vi "DriveStateController2.vi"(1 "Selected State (In)":string) -> (0 "Selected State (Out)":string)   [LabVIEW 2019]
doc: "This VI performs all of the calculations and decisions related to the swerve drive."
uses:
  dsinstructions.vi
  outputs.vi
  sensors.vi
  dsdata.vi
  constants.vi
panel:
  out "Heading Control":bool
  in  "Heading Lock Strafe Deadband (ft/s)":dbl=2.0
  in  "PID Tuning Heading Lock":T1={"Kp"=0.007, "Ki"=0.03, "Kd"=0.0015, "N-Diff"=5, "N-Int"=10, "Int Error Window"=30.0, "Max Ouput"=1.0, "Min Output"=-1.0} {"Int Error Window" min=0.0; "N-Int" min=2; "N-Diff" min=2; "Kd" min=0.0; "Ki" min=0.0; "Kp" min=0.0}
  in  "Manually Disable Heading Lock":bool
  in  "PID Tuning Feeder Station":T1={"Kp"=0.01, "Ki"=0.01, "Kd"=9e-05, "N-Diff"=10, "N-Int"=10, "Int Error Window"=30.0, "Max Ouput"=1.0, "Min Output"=-1.0} {"Int Error Window" min=0.0; "N-Int" min=2; "N-Diff" min=2; "Kd" min=0.0; "Ki" min=0.0; "Kp" min=0.0}
  out "Heading Controller Summary":T2(graph)
  in  "PID Tuning Auto Targeting":T1={"Kp"=0.01, "Ki"=0.01, "Kd"=9e-05, "N-Diff"=10, "N-Int"=10, "Int Error Window"=30.0, "Max Ouput"=1.0, "Min Output"=-1.0} {"Int Error Window" min=0.0; "N-Int" min=2; "N-Diff" min=2; "Kd" min=0.0; "Ki" min=0.0; "Kp" min=0.0}
  in  "Manual Fudge Factor (deg)":dbl=5.0
  in  "Plot Heading PID":bool
  in  "Rotation Scaling":dbl[](array[slide])=[2.5, 2.5, 2.5, 2.5] min=1.0 max=4.0 scale=1.0..4.0
  in  "Strafe Scaling":dbl[](array[slide])=[3.0, 2.0, 2.0, 2.0] min=1.0 max=4.0 scale=1.0..4.0
  in  "Rotation Deadband":dbl[](array[slide])=[0.15, 0.15, 0.15, 0.15] min=0.0 max=0.4 scale=0.0..0.4
  in  "Strafe Deadband":dbl[](array[slide])=[0.08, 0.08, 0.08, 0.08] min=0.0 max=0.4 scale=0.0..0.4
  in  "Sync Driver Profile":bool
  out "Current_Driver":string
  in  "Zero Wheels":bool
  in  "Best Angle Hysteresis (deg)":dbl=20.0 format="%#_13g"
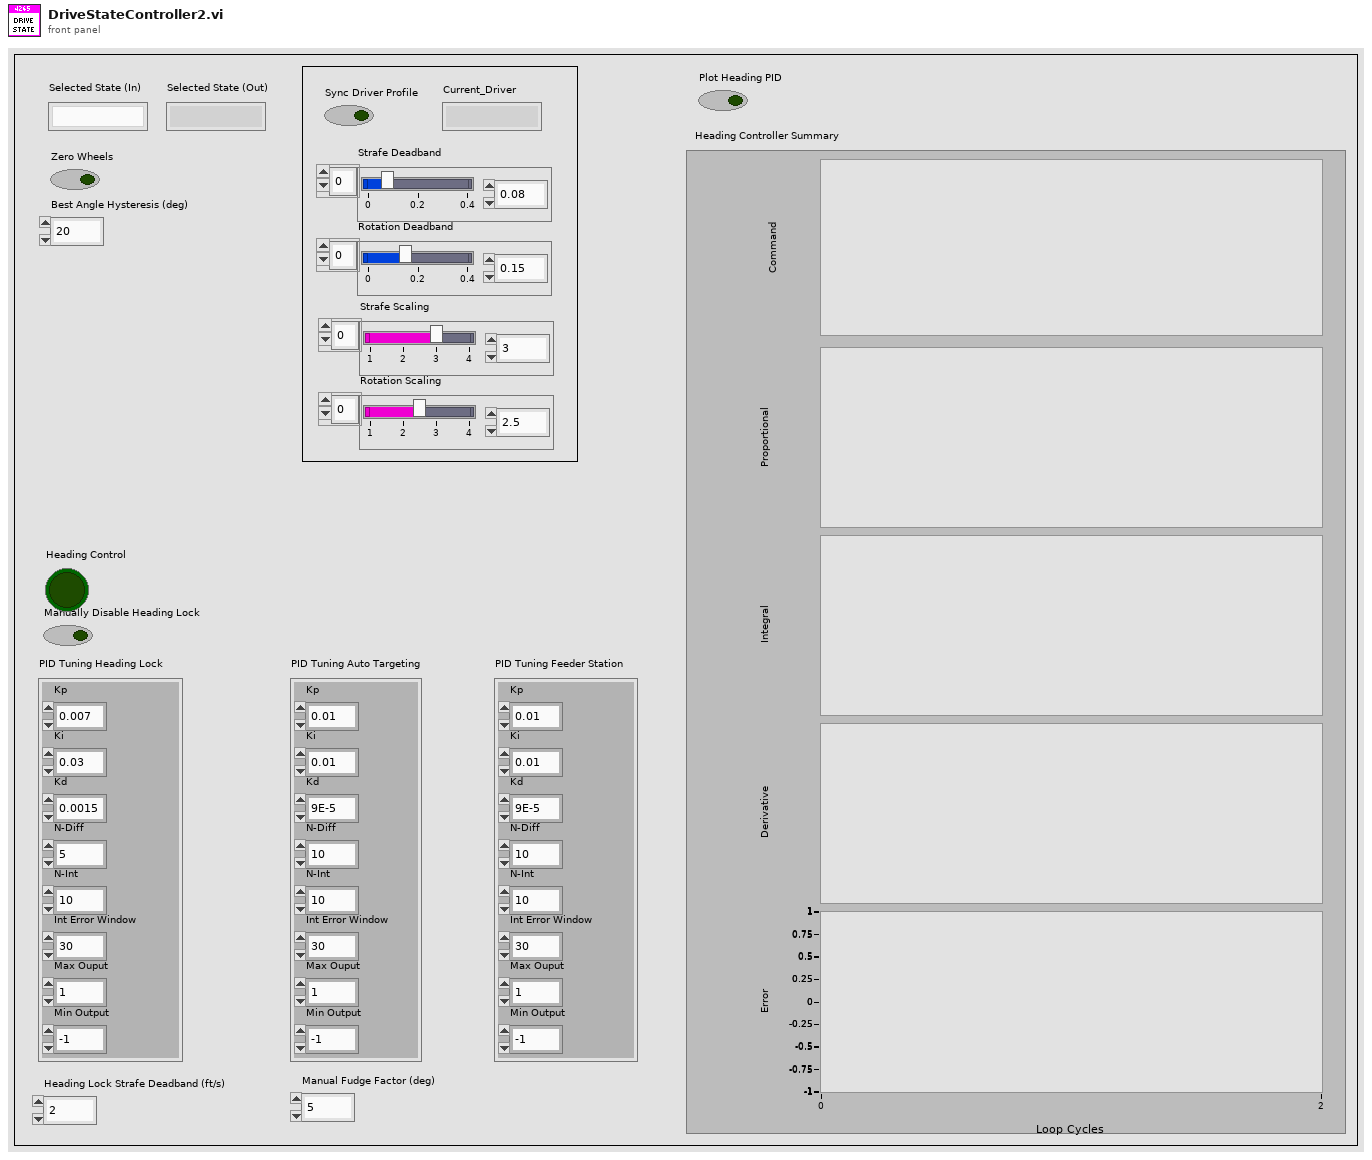
[diagram p1: front panel]
types:
  T1 = cluster{"Kp":dbl, "Ki":dbl, "Kd":dbl, "N-Diff":i32, "N-Int":i32, "Int Error Window":dbl, "Max Ouput":dbl, "Min Output":dbl}
  T2 = cluster{"Command":dbl, "Proportional":dbl, "Integral":dbl, "Derivative":dbl, "Goal":dbl}
  T3 = enum16{"Driver Control", "Auto Targeting", "Feeder Station"}
  T4 = enum16{"Center", "Module 0", "Module 1", "Module 2", "Module 3"}
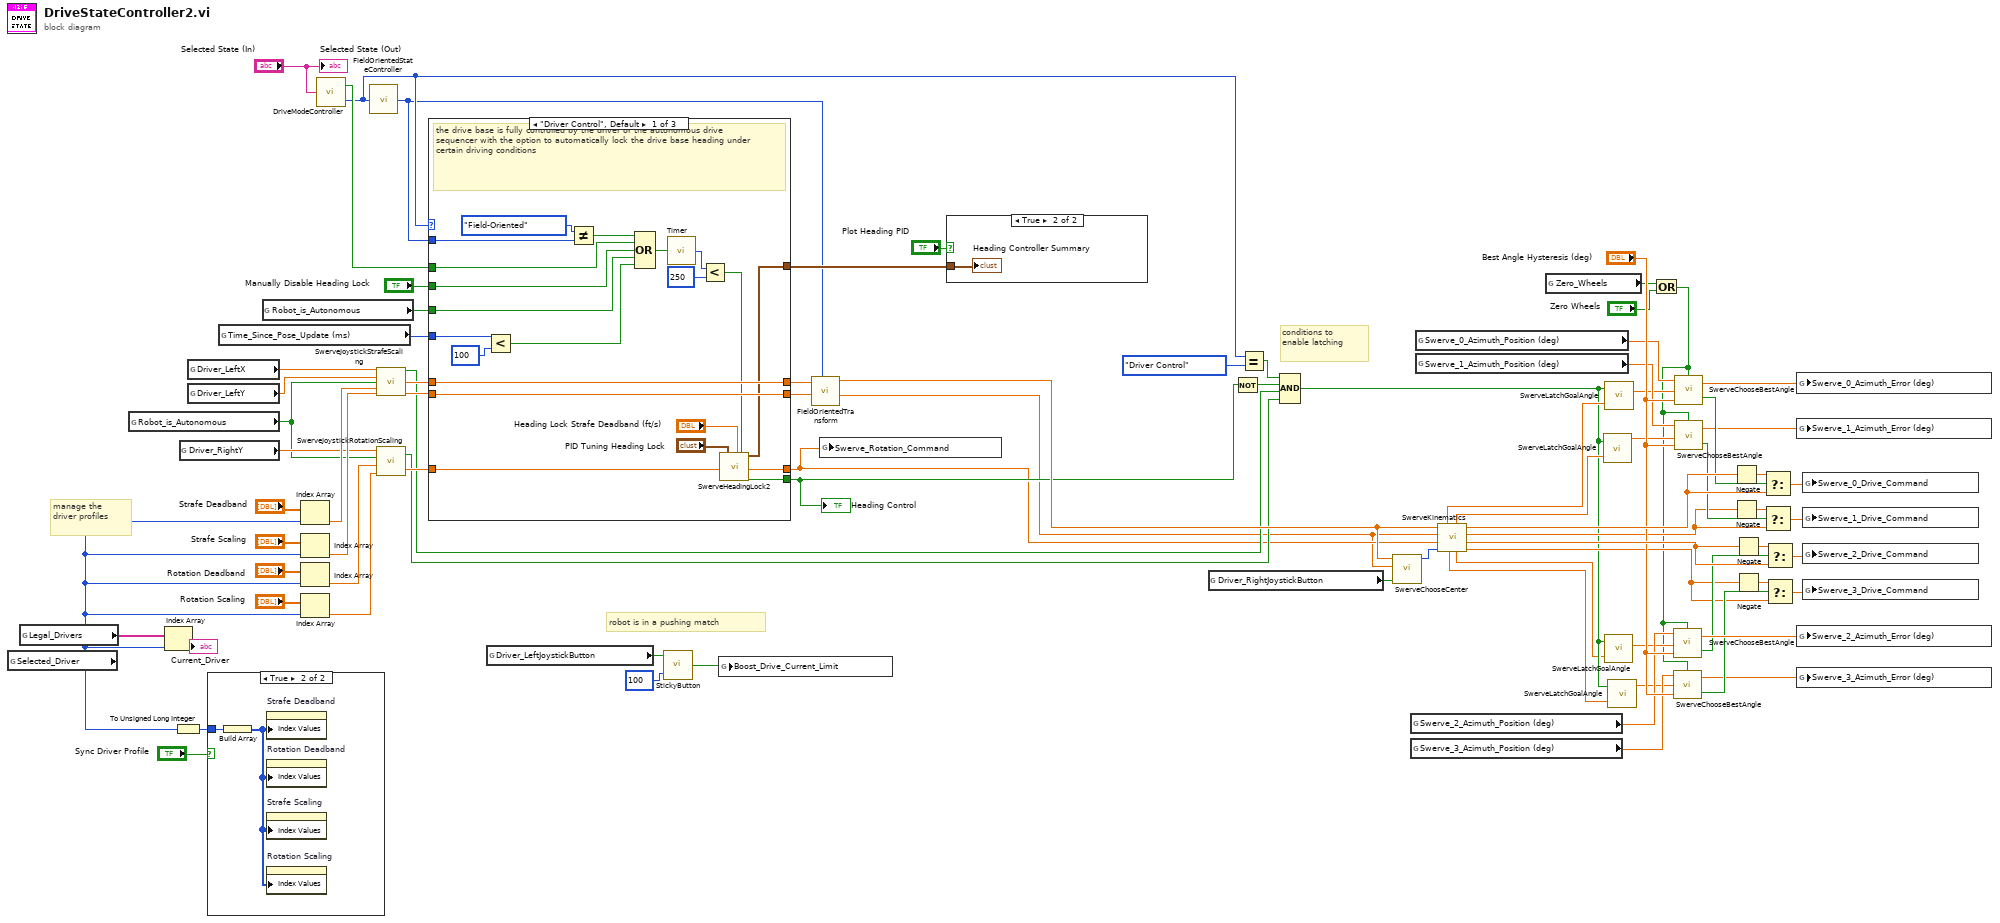
[diagram p0: block diagram]
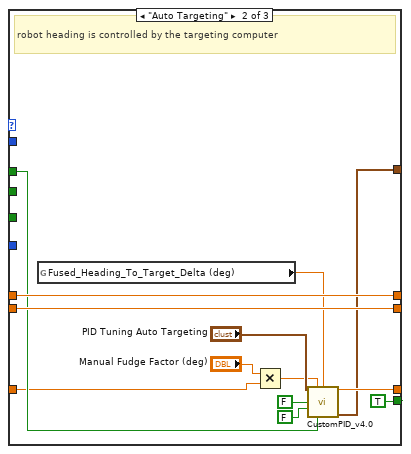
[diagram p3: hidden frame]
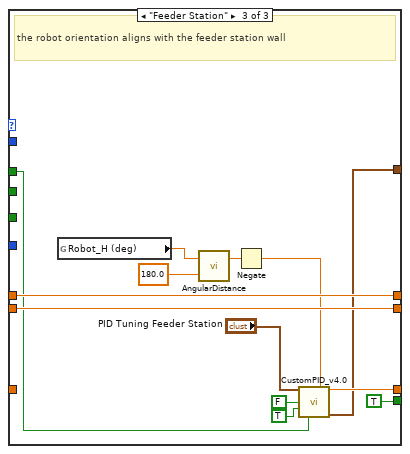
[diagram p4: hidden frame]
diagram:
  # "robot is in a pushing match"
  # "conditions to\nenable latching"
  # "manage the\ndriver profiles"
  n1 = global read "dsdata.vi" "Selected_Driver"() -> (w34:i32)
  n2 = global read "constants.vi" "Legal_Drivers"() -> (w40:string[])
  n3 = global read "dsdata.vi" "Robot_is_Autonomous"() -> (w15:bool)
  n4 = Index Array(array=w40, index=w34) -> (element=→"Current_Driver":string)
  n5 = To Unsigned Long Integer(number=w34) -> (unsigned 32bit integer=w46:u32)
  n6 = global read "dsinstructions.vi" "Driver_RightY"() -> (w16:dbl)
  n7 = global read "dsinstructions.vi" "Driver_LeftX"() -> (w23:dbl)
  n8 = global read "dsinstructions.vi" "Driver_LeftY"() -> (w22:dbl)
  n9 = case shown="True" "Sync Driver Profile" {
    tunnel: w46 -> [_ w84]
    frame False {
    }
    frame True {
      n10 = Build Array(w84) -> (w83:u32[])
      n11 = property on="Strafe Deadband" class="Arr (strict)"("Index Values"=w83) -> ()  [unwired: 2 in, 2 out]
      n12 = property on="Rotation Deadband" class="Arr (strict)"("Index Values"=w83) -> ()  [unwired: 2 in, 2 out]
      n13 = property on="Strafe Scaling" class="Arr (strict)"("Index Values"=w83) -> ()  [unwired: 2 in, 2 out]
      n14 = property on="Rotation Scaling" class="Arr (strict)"("Index Values"=w83) -> ()  [unwired: 2 in, 2 out]
    }
  }
  n15 = global read "sensors.vi" "Time_Since_Pose_Update (ms)"() -> (w33:u32)
  n16 = global read "dsdata.vi" "Robot_is_Autonomous"() -> (w32:bool)
  n17 = Index Array(array="Strafe Deadband", index=w34) -> (element=w19:dbl)
  n18 = Index Array(array="Strafe Scaling", index=w34) -> (element=w18:dbl)
  n19 = Index Array(array="Rotation Deadband", index=w34) -> (element=w14:dbl)
  n20 = Index Array(array="Rotation Scaling", index=w34) -> (element=w13:dbl)
  n21 = call "DriveModeController.vi"("Selected State (In)"="Selected State (In)") -> ("Drive Mode Change"=w30:bool, "Drive Mode"=w5:T3)
  n22 = call "FieldOrientedStateController.vi"("Drive Mode"=w5) -> ("Orientation Mode"=w2:enum16{"Robot-Oriented", "Field-Oriented"})
  n23 = call "SwerveJoystickStrafeScaling.vi"("Raw Joystick X"=w23, "Raw Joystick Y"=w22, "Auto Control"=w15, "Strafe Deadband"=w19, "Strafe Scaling"=w18) -> ("In Deadband"=w9:bool, "Scaled Joystick X"=w21:dbl, "Scaled Joystick Y"=w20:dbl)  [unwired: 8 in]
  n24 = call "SwerveJoystickRotationScaling.vi"("Rotation Scaling"=w13, "Rotation Deadband"=w14, "Auto Control"=w15, "Raw Joystick Rotation"=w16) -> ("Scaled Joystick Rotation"=w17:dbl, "In Deadband"=w10:bool)
  n25 = case shown="\"Driver Control\", Default" w5 {
    tunnel: [w101 w117 w129] -> w1
    tunnel: [w100 w118 w127] -> w59
    tunnel: w21 -> [w100 w118 w127]
    tunnel: w20 -> [w101 w117 w129]
    tunnel: w17 -> [w93 w107 _]
    tunnel: [w94 w109 w126] -> w8
    tunnel: [w99 TRUE ("auto rot control") TRUE ("auto rot control")] -> w11
    tunnel: w2 -> [w102 _ _]
    tunnel: w32 -> [w97 _ _]
    tunnel: w30 -> [w90 w112 w122]
    tunnel: w33 -> [w105 _ _]
    tunnel: [w96 w108 w121] -> w31
    tunnel: "Manually Disable Heading Lock" -> [w95 _ _]
    frame "Driver Control", Default {
      # "the drive base is fully controlled by the driver or the autonomous drive sequencer with the option to automatically lock the drive base heading under certain driving conditions"
      n26 = Less?(x=w105, y=u32 100) -> (x < y?=w98:bool)
      n27 = Not Equal?(x=enum16{"Robot-Oriented", "Field-Oriented"}."Field-Oriented" ("Orientation Mode"), y=w102) -> (x != y?=w89:bool)
      n28 = Compound Arithmetic op=OR(w89, w90, w95, w97, w98) -> (w87:bool)
      n29 = call "Timer.vi"("Reset Timer"=w87) -> ("Time (ms)"=w88:u32)
      n30 = Less?(x=w88, y=u32 250) -> (x < y?=w85:bool)
      n31 = call "SwerveHeadingLock2.vi"("Driver Rotation Joystick"=w93, "PID Tuning Parameters"="PID Tuning Heading Lock", "Heading Lock Strafe Deadband (ft/s)"="Heading Lock Strafe Deadband (ft/s)", "External Disables"=w85) -> ("Controller Summary"=w96:T2, "Joystick Rotation"=w94:dbl, "Heading Lock"=w99:bool)  [unwired: 13 in]
    }
    frame "Auto Targeting" {
      # "robot heading is controlled by the targeting computer"
      n32 = global read "sensors.vi" "Fused_Heading_To_Target_Delta (deg)"() -> (w113:dbl)
      n33 = Multiply(x="Manual Fudge Factor (deg)", y=w107) -> (x*y=w114:dbl)
      n34 = call "CustomPID_v4.0.vi"("PID Tuning Parameters"="PID Tuning Auto Targeting", "Goal"=w114, "Process Variable"=w113, "Reset on Goal Change ?"=FALSE, "Use Custom Error Calculation ?"=FALSE, "Reinit"=w112) -> ("Command"=w109:dbl, "Controller Summary"=w108:T2)  [unwired: 6 in, 2 out]
    }
    frame "Feeder Station" {
      # "the robot orientation aligns with the feeder station wall"
      n35 = global read "sensors.vi" "Robot_H (deg)"() -> (w131:dbl)
      n36 = call "AngularDistance.vi"("Goal Angle (deg) [0,360]"=180.0, "Current Angle (deg) [-Inf,+Inf]"=w131) -> ("Signed Angular Distance (deg) [-180,+180]"=w120:dbl)  [unwired: 1 out]
      n37 = Negate(x=w120) -> (-x=w119:dbl)
      n38 = call "CustomPID_v4.0.vi"("PID Tuning Parameters"="PID Tuning Feeder Station", "Custom Error Calculation"=w119, "Reset on Goal Change ?"=FALSE, "Use Custom Error Calculation ?"=TRUE, "Reinit"=w122) -> ("Command"=w126:dbl, "Controller Summary"=w121:T2)  [unwired: 7 in, 2 out]
    }
  }
  "Heading Control" <- w11
  n39 = global read "dsinstructions.vi" "Driver_LeftJoystickButton"() -> (w26:bool)
  n40 = call "StickyButton.vi"("Time threshold (ms)"=u32 100 ("y"), "Button Input"=w26) -> ("Sticky Button"=w24:bool)
  n41 = global write "outputs.vi" "Boost_Drive_Current_Limit"(w24) -> ()
  n42 = call "FieldOrientedTransform.vi"("Orientation Mode"=w2, "Joystick Y"=w1, "Joystick X"=w59) -> ("Joystick Y'"=w3:dbl, "Joystick X'"=w12:dbl)  [unwired: 7 in]
  n43 = global write "outputs.vi" "Swerve_Rotation_Command"(w8) -> ()
  n44 = case shown="True" "Plot Heading PID" {
    tunnel: w31 -> [_ w132]
    frame False {
    }
    frame True {
      "Heading Controller Summary" <- w132
    }
  }
  n45 = global read "dsinstructions.vi" "Driver_RightJoystickButton"() -> (w29:bool)
  n46 = Not(x=w11) -> (.not. x?=w7:bool)
  n47 = Equal?(x=w5, y=T3."Driver Control" ("x")) -> (x = y?=w6:bool)
  n48 = Compound Arithmetic op=AND(w6, w7, w9, w10) -> (w37:bool)
  n49 = call "SwerveChooseCenter.vi"("Defensive Driving Trigger"=w29, "Joystick Y"=w3, "Joystick X"=w12) -> ("Center Choice"=w28:T4)  [unwired: 6 in]
  n50 = global read "sensors.vi" "Swerve_2_Azimuth_Position (deg)"() -> (w74:dbl)
  n51 = global read "sensors.vi" "Swerve_3_Azimuth_Position (deg)"() -> (w60:dbl)
  n52 = global read "sensors.vi" "Swerve_0_Azimuth_Position (deg)"() -> (w62:dbl)
  n53 = global read "sensors.vi" "Swerve_1_Azimuth_Position (deg)"() -> (w61:dbl)
  n54 = call "SwerveKinematics.vi"("Rotation Center Choice"=w28, "Joystick Rotation"=w8, "Joystick Y"=w3, "Joystick X"=w12) -> ("Module 3 Velocity (ul)"=w51:dbl, "Module 2 Velocity (ul)"=w80:dbl, "Module 1 Velocity (ul)"=w52:dbl, "Module 0 Velocity (ul)"=w79:dbl, "Module 2 Angle (deg)"=w36:dbl, "Module 1 Angle (deg)"=w53:dbl, "Module 3 Angle (deg)"=w35:dbl, "Module 0 Angle (deg)"=w58:dbl)
  n55 = global read "dsdata.vi" "Zero_Wheels"() -> (w50:bool)
  n56 = call "SwerveLatchGoalAngle.vi"("Raw Goal Angle"=w53, "In Deadband"=w37) -> ("Latched Goal Angle"=w56:dbl)
  n57 = call "SwerveLatchGoalAngle.vi"("Raw Goal Angle"=w36, "In Deadband"=w37) -> ("Latched Goal Angle"=w55:dbl)
  n58 = call "SwerveLatchGoalAngle.vi"("Raw Goal Angle"=w58, "In Deadband"=w37) -> ("Latched Goal Angle"=w57:dbl)
  n59 = call "SwerveLatchGoalAngle.vi"("Raw Goal Angle"=w35, "In Deadband"=w37) -> ("Latched Goal Angle"=w54:dbl)
  n60 = Or(x=w50, y="Zero Wheels") -> (x .or. y?=w49:bool)
  n61 = call "SwerveChooseBestAngle.vi"("Zero Wheels"=w49, "Hysteresis (deg)"="Best Angle Hysteresis (deg)", "Goal Angle (deg) [-180,+180]"=w55, "Current Angle (deg) [-180,+180]"=w74) -> ("Invert Speed  Motor (?)"=w76:bool, "Angular Distance (deg)"=w77:dbl)
  n62 = call "SwerveChooseBestAngle.vi"("Zero Wheels"=w49, "Hysteresis (deg)"="Best Angle Hysteresis (deg)", "Goal Angle (deg) [-180,+180]"=w54, "Current Angle (deg) [-180,+180]"=w60) -> ("Invert Speed  Motor (?)"=w75:bool, "Angular Distance (deg)"=w65:dbl)
  n63 = call "SwerveChooseBestAngle.vi"("Zero Wheels"=w49, "Hysteresis (deg)"="Best Angle Hysteresis (deg)", "Goal Angle (deg) [-180,+180]"=w57, "Current Angle (deg) [-180,+180]"=w62) -> ("Invert Speed  Motor (?)"=w69:bool, "Angular Distance (deg)"=w67:dbl)
  n64 = call "SwerveChooseBestAngle.vi"("Zero Wheels"=w49, "Hysteresis (deg)"="Best Angle Hysteresis (deg)", "Goal Angle (deg) [-180,+180]"=w56, "Current Angle (deg) [-180,+180]"=w61) -> ("Invert Speed  Motor (?)"=w68:bool, "Angular Distance (deg)"=w66:dbl)
  n65 = Negate(x=w79) -> (-x=w73:dbl)
  n66 = Negate(x=w52) -> (-x=w71:dbl)
  n67 = Negate(x=w80) -> (-x=w82:dbl)
  n68 = Negate(x=w51) -> (-x=w64:dbl)
  n69 = Select(t=w73, s=w69, f=w79) -> (s? t:f=w72:dbl)
  n70 = Select(t=w71, s=w68, f=w52) -> (s? t:f=w70:dbl)
  n71 = Select(t=w82, s=w76, f=w80) -> (s? t:f=w81:dbl)
  n72 = Select(t=w64, s=w75, f=w51) -> (s? t:f=w63:dbl)
  n73 = global write "outputs.vi" "Swerve_0_Azimuth_Error (deg)"(w67) -> ()
  n74 = global write "outputs.vi" "Swerve_1_Azimuth_Error (deg)"(w66) -> ()
  n75 = global write "outputs.vi" "Swerve_2_Azimuth_Error (deg)"(w77) -> ()
  n76 = global write "outputs.vi" "Swerve_3_Azimuth_Error (deg)"(w65) -> ()
  n77 = global write "outputs.vi" "Swerve_0_Drive_Command"(w72) -> ()
  n78 = global write "outputs.vi" "Swerve_1_Drive_Command"(w70) -> ()
  n79 = global write "outputs.vi" "Swerve_2_Drive_Command"(w81) -> ()
  n80 = global write "outputs.vi" "Swerve_3_Drive_Command"(w63) -> ()
  "Selected State (Out)" <- "Selected State (In)"
